vi "Read Impulsator.vi"(8 "error in (no error)":errorcluster, 11 "HE_reg in":refnum<class "HE_reg.lvclass">) -> (0 "error out":errorcluster, 2 "Impulsator":refnum<class "Impulsator.lvclass">, 3 "HE_reg out":refnum<class "HE_reg.lvclass">)   [LabVIEW 2019, in "Heating.lvlib" / "HE_reg.lvclass"]
uses:
  HE_reg.lvclass
  Transform/Impulsator.lvclass
  HE_reg.lvclass/HE_reg.ctl
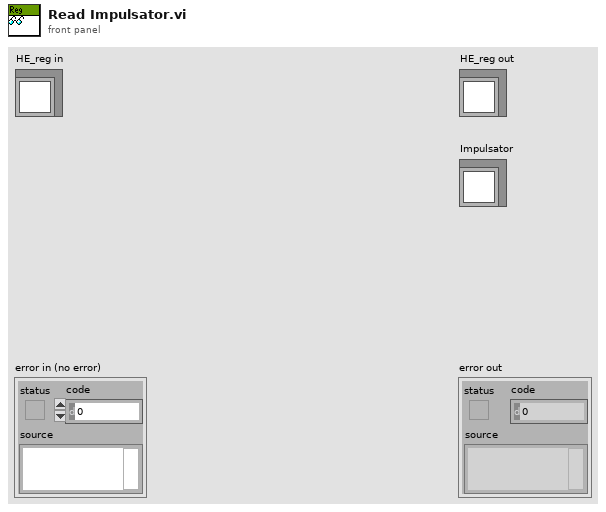
[diagram p1: front panel]
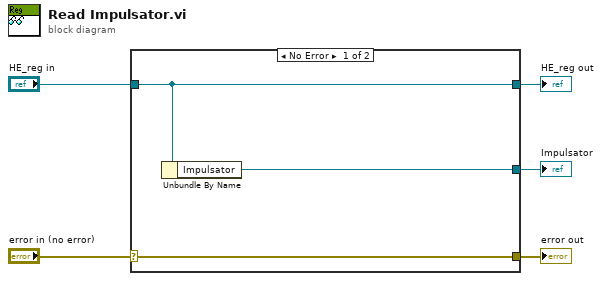
[diagram p0: block diagram]
diagram:
  n1 = case shown="No Error" "error in (no error)" {
    selector: "error in (no error)" -> [w8 w9]
    tunnel: [w8 w9] -> w4
    tunnel: [w7 w10] -> w2
    tunnel: "HE_reg in" -> [w7 w10]
    tunnel: [w6 _] -> w1
    frame No Error {
      n2 = Unbundle By Name(w7) -> ("Impulsator"=w6:refnum<class "Impulsator.lvclass">)
    }
    frame Error {
    }
  }
  "error out" <- w4
  "HE_reg out" <- w2
  "Impulsator" <- w1
